vi "Send LastAck.vi"(8 "error in (no error)":errorcluster, 11 "Module in":refnum<class "Module.lvclass">) -> (0 "error out":errorcluster)   [LabVIEW 2020, in "Volatus.lvlib" / "Module.lvclass"]
uses:
  Module.lvclass
  LastAck.ctl
  Module.lvclass/Module.ctl
  MessageQ/MessageQ.lvclass/MessageQ.ctl
  MessageQ/MessageQ.lvclass
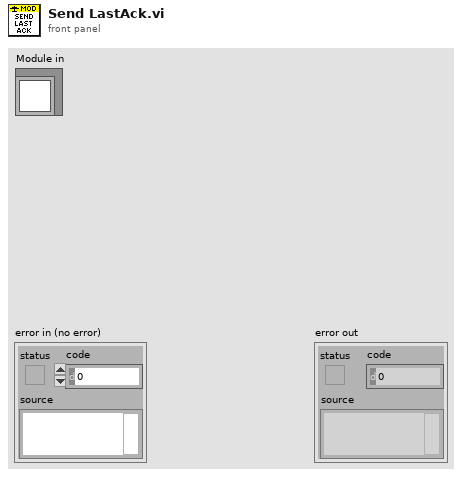
[diagram p1: front panel]
types:
  T1 = typedef "Volatus.lvlib/Module.lvclass/LastAck.ctl" = cluster{"Module":refnum<class "Module.lvclass">}
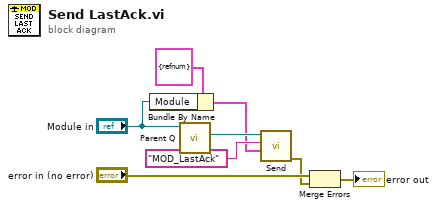
[diagram p0: block diagram]
diagram:
  n1 = Bundle By Name(cluster=T1 {"Module"=refnum} ("LastAck"), "Module"="Module in") -> (w3:T1)
  n2 = call "Parent Q.vi"("Module in"="Module in") -> ("Parent Q"=w5:refnum<class "MessageQ.lvclass">)  [unwired: 9 in, 1 out]
  n3 = call "Send.vi"("Data"=w3, "ID"="MOD_LastAck", "MessageQ in"=w5) -> ("error out"=w1:errorcluster)  [unwired: 7 in, 1 out]
  n4 = Merge Errors("error in (no error)", w1) -> (→"error out":errorcluster)
